vi "Subtask 1.vi"() -> ()   [LabVIEW 2016, in "Test.lvrbt"]
uses:
  Test.lvrbt
  <vilib>/NXT/Block Support/NXT_OutputPort.ctl
  <vilib>/NXT/Block Support/NXT_InputPort.ctl
  <vilib>/NXT/Dual Mode Library/Motors/ResetMotor.vi
  <vilib>/NXT/Dual Mode Library/Waits/Wait_Num(msec).vi
  <vilib>/NXT/Dual Mode Library/Display/drawText.vi
  <vilib>/NXT/Dual Mode Library/Sensors/EV3_Color_Reflect.vi
  <vilib>/NXT/Dual Mode Library/Sensors/Touch_Pressed.vi
  <vilib>/NXT/Dual Mode Library/Sensors/EV3_Ultrasonic_CM.vi
  <vilib>/NXT/Dual Mode Library/Motors/Rotation.vi
  <vilib>/NXT/NXTIO Xnodes/NXTIONodeSubVIs/NXTMoveMotors.vi
  <vilib>/NXT/NXTIO Xnodes/NXTIONodeSubVIs/NXTMotorRunDistance.vi
  <vilib>/NXT/Dual Mode Library/Display/drawNumber.vi
  <vilib>/NXT/NXTIO Xnodes/NXTIONodeSubVIs/NXTMotorSteeringOn.vi
  <vilib>/NXT/NXTIO Xnodes/AddressXNode/NXTIOAddress.xnode
  <vilib>/NXT/Subs/LVHSConnector.ctl
  <vilib>/NXT/NXTIO Xnodes/NXTIOXNode/NXTIO.xnode
  <vilib>/NXT/LegoClasses/BrickReference/BrickReference.lvclass
panel:
  out "kD":dbl(graph)
  out "kI":dbl(graph)
  out "kP":sgl(graph)
  out "Combined":dbl(graph)
  out "Power Sum":dbl
  out "power":dbl
  out "rotation":dbl
  out "button":bool
  out "Distance":dbl
  out "Box Number":dbl
  out "Zone Detector":dbl
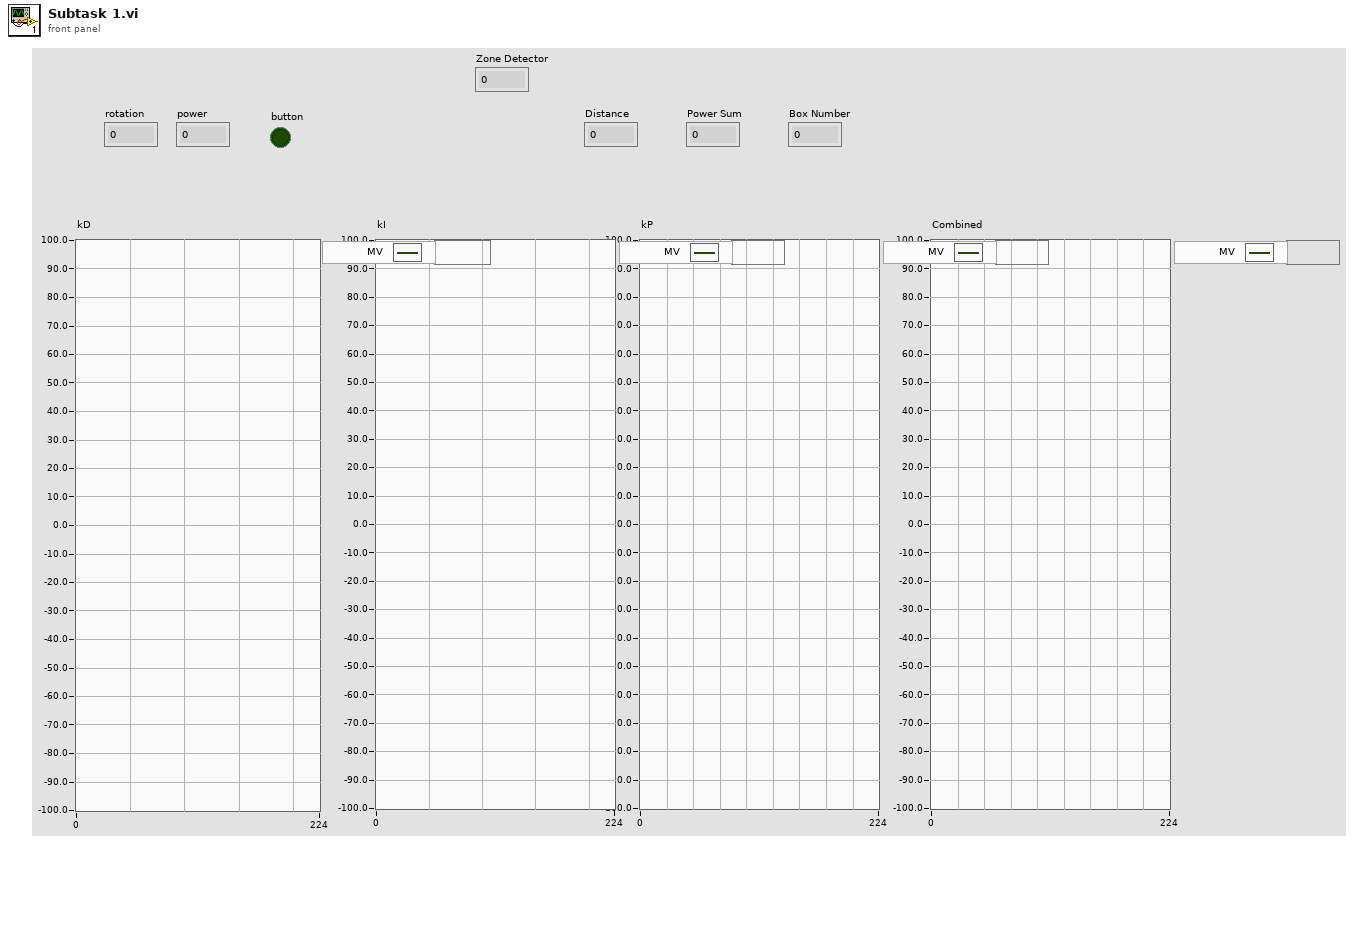
[diagram p1: front panel]
types:
  T1 = typedef "NXT_OutputPort.ctl" = u8
  T2 = typedef "NXT_InputPort.ctl" = u32
  T3 = typedef "LVHSConnector.ctl" = refnum<class "BrickReference.lvclass">
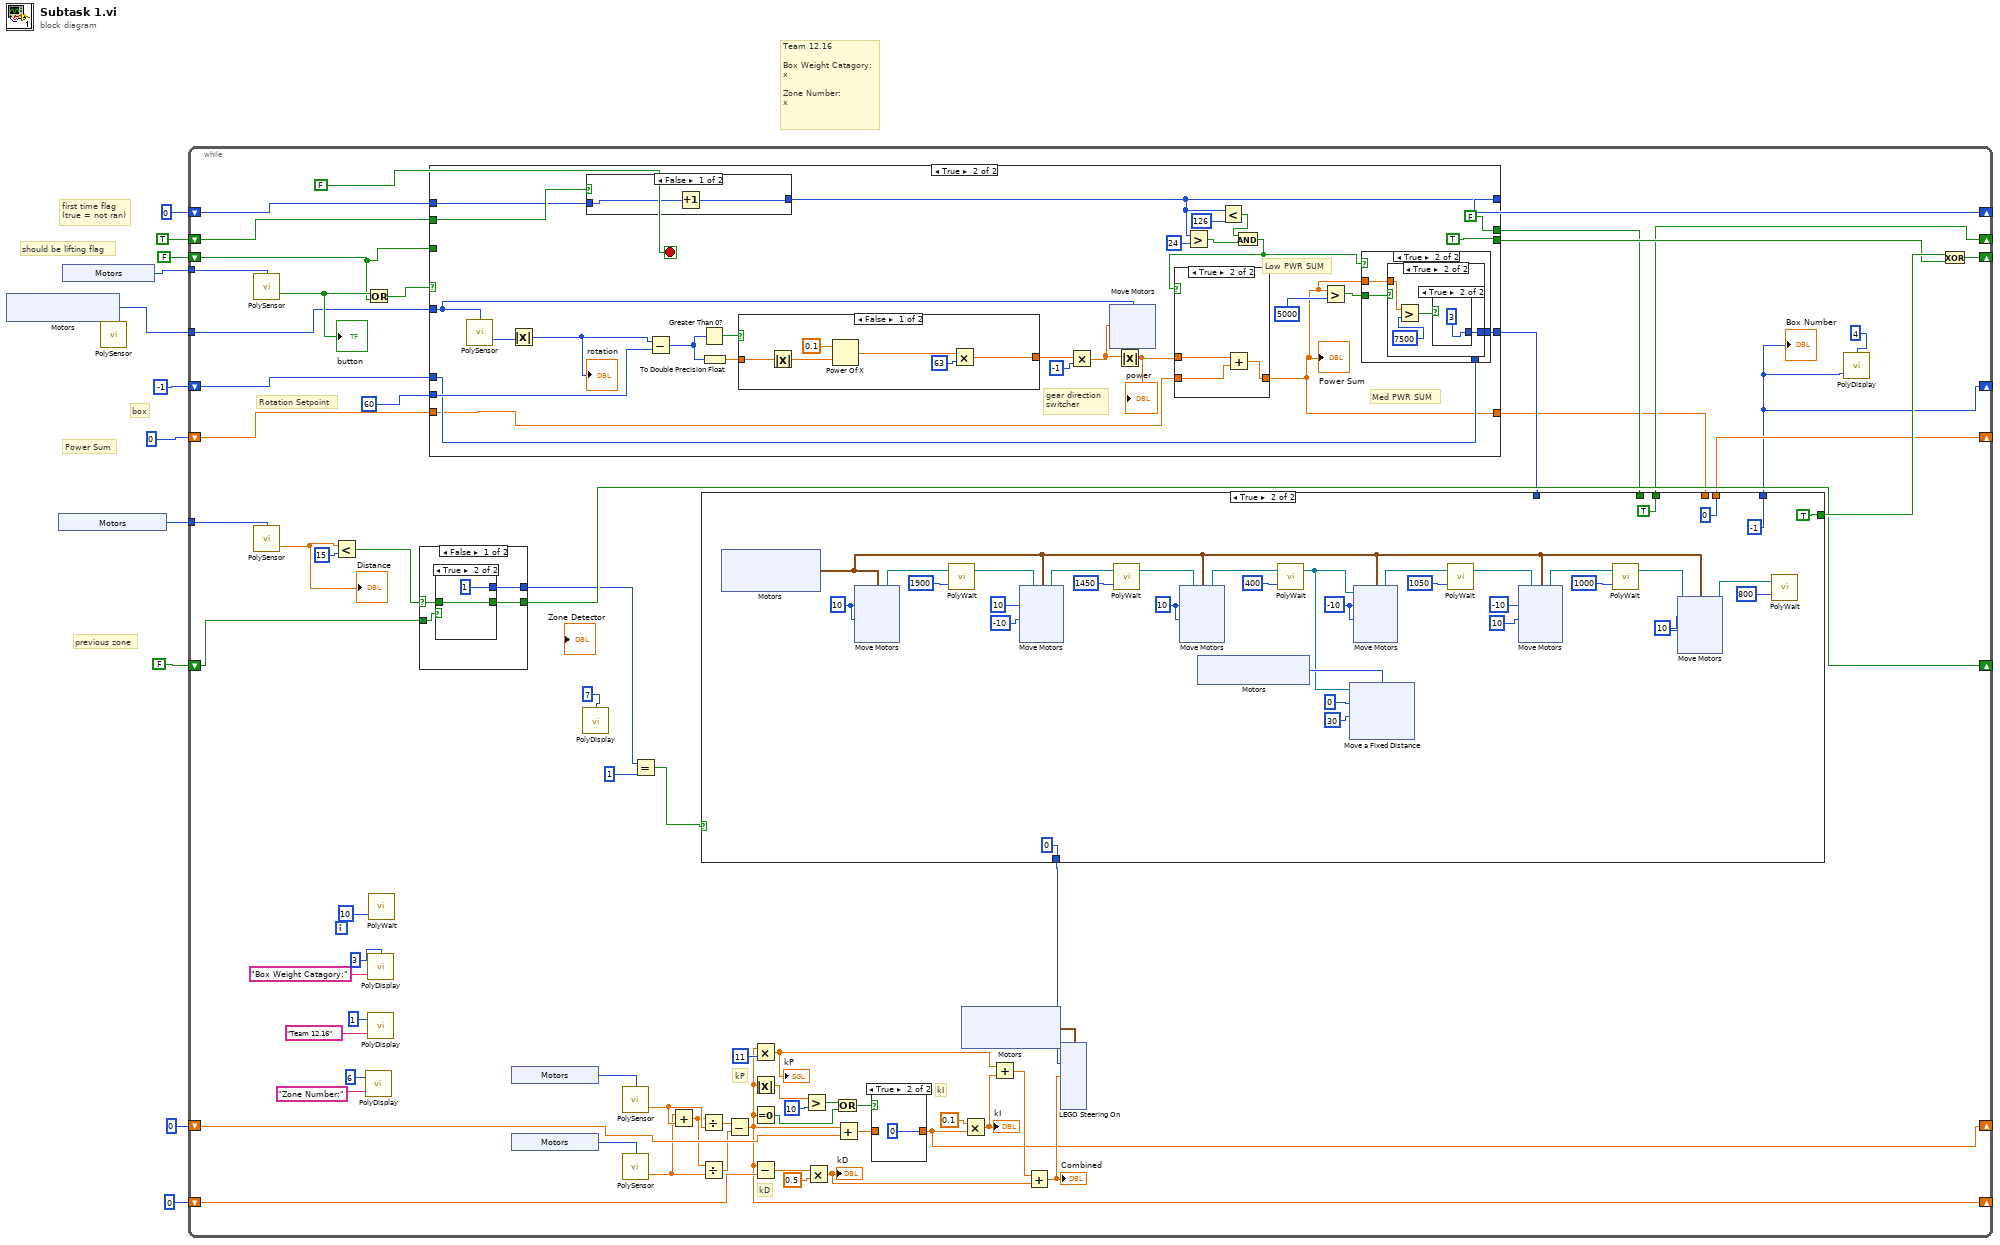
[diagram p0: block diagram]
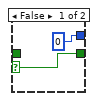
[diagram p2: hidden frame]
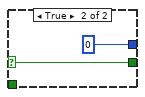
[diagram p3: hidden frame]
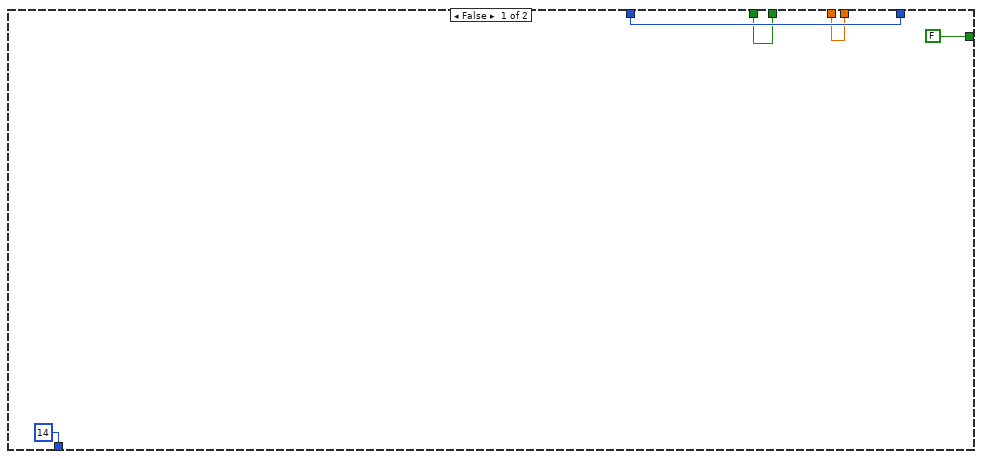
[diagram p4: hidden frame]
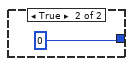
[diagram p6: hidden frame]
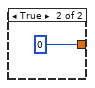
[diagram p8: hidden frame]
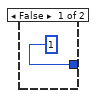
[diagram p10: hidden frame]
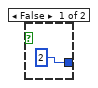
[diagram p11: hidden frame]
diagram:
  # "box"
  # "previous zone"
  # "Team 12.16\n\nBox Weight Catagory:\nx\n\nZone Number:\nx"
  # "should be lifting flag"
  # "first time flag\n(true = not ran)"
  # "Power Sum"
  n1 = xnode "Motors"() -> ("Motor"=w1:T1)
  n2 = xnode "Motors"() -> ("Sensor"=w8:T2)
  n3 = xnode "Motors"() -> ("Sensor"=w7:T2)
  n4 = call-poly <vilib>:"PolySensor.vi"("Port (All Ports)"=w1) -> ()  [unwired: 3 in, 1 out]
  n5 = while {
    shift-right: [w50] -> _
    shift-left: 0 -> [w77]
    shift-right: [w51] -> _
    shift-left: 0 -> [w76]
    tunnel: w1 -> [w32]
    shift-right: [w48] -> _
    shift-left: FALSE -> [w44]
    tunnel: w8 -> [w41]
    tunnel: w7 -> [w42]
    shift-right: [w14] -> _
    shift-left: -1 -> [w40]
    shift-right: [w18] -> _
    shift-left: TRUE -> [w39]
    shift-right: [w16] -> _
    shift-left: 0 -> [w36]
    shift-right: [w34] -> _
    shift-left: u32 0 ("Time (100 msec)") -> [w35]
    shift-right: [w21] -> _
    shift-left: FALSE -> [w22]
    stop <- FALSE stop-if-true
    # "Rotation Setpoint"
    # "kD"
    # "kI"
    # "kP"
    n6 = call-poly <vilib>:"PolySensor.vi"("Port (Port 1)"=w42) -> ("Yes / No"=w53:bool)  [unwired: 2 in, 1 out]
    "button" <- w53
    n7 = call-poly <vilib>:"PolySensor.vi"("Port (Port 1)"=w41) -> ("Centimeters"=w38:sgl)  [unwired: 2 in, 1 out]
    "Distance" <- w38
    n8 = Less?(x=w38, y=15) -> (x < y?=w23:bool)
    n9 = call-poly <vilib>:"PolyDisplay.vi"("Text"="Zone Number:", "Line"=6 ("number")) -> ()  [unwired: 2 in, 1 out]
    n10 = Or(x=w53, y=w44) -> (x .or. y?=w52:bool)
    n11 = call-poly <vilib>:"PolyDisplay.vi"("Text"="Box Weight Catagory:", "Line"=3 ("number")) -> ()  [unwired: 2 in, 1 out]
    n12 = call-poly <vilib>:"PolyDisplay.vi"("Text"="Team 12.16", "Line"=1 ("number")) -> ()  [unwired: 2 in, 1 out]
    n13 = call-poly <vilib>:"PolyWait.vi"("Time (100 msec)"=u32 10) -> ()  [unwired: 3 in, 1 out]
    n14 = case shown="False" w23 {
      selector: w23 -> [w80 w88]
      tunnel: w22 -> [w82 _]
      tunnel: [w81 w88] -> w21
      tunnel: [w79 0] -> w13
      frame False {
        n15 = case shown="True" w82 {
          selector: w82 -> [w84 _]
          tunnel: [w84 w86] -> w81
          tunnel: w80 -> [_ w86]
          tunnel: [0 1] -> w79
          frame False {
          }
          frame True {
          }
        }
      }
      frame True {
      }
    }
    n16 = case shown="True" w52 {
      tunnel: w32 -> [_ w219]
      tunnel: 60 -> [_ w218]
      tunnel: [w192 TRUE] -> w45
      tunnel: w44 -> [w192 _]
      tunnel: [w191 w214] -> w19
      tunnel: w40 -> [w191 w213]
      tunnel: [w190 FALSE] -> w17
      tunnel: w39 -> [w190 w206]
      tunnel: w36 -> [w189 w208]
      tunnel: [w189 w207] -> w15
      tunnel: w35 -> [w188 w205]
      tunnel: [w188 w204] -> w34
      frame False {
      }
      frame True {
        # "gear direction\nswitcher"
        # "Med PWR SUM"
        # "Low PWR SUM"
        n17 = call-poly <vilib>:"PolySensor.vi"("Port (Port A)"=w219) -> ("Angle of Rotation"=w200:i32)  [unwired: 2 in, 1 out]
        n18 = Absolute Value(x=w200) -> (abs(x)=w199:i32)
        "rotation" <- w199
        n19 = case shown="False" w206 {
          tunnel: [w220 u32 0 ("Time (100 msec)")] -> w204
          tunnel: w205 -> [w221 _]
          frame False {
            n20 = Increment(x=w221) -> (x+1=w220:u32)
          }
          frame True {
          }
        }
        n21 = Subtract(x=w199, y=w218) -> (x-y=w212:i32)
        n22 = Greater Than 0?(x=w212) -> (x > 0?=w211:bool)
        n23 = To Double Precision Float(number=w212) -> (double precision float=w210:dbl)
        n24 = case shown="False" w211 {
          tunnel: [w229 0] -> w196
          tunnel: w210 -> [w228 _]
          frame False {
            n25 = Absolute Value(x=w228) -> (abs(x)=w227:dbl)
            n26 = Power Of X(1:w227, 2:0.1) -> (0:w230:dbl)
            n27 = Multiply(x=w230, y=63) -> (x*y=w229:dbl)
          }
          frame True {
          }
        }
        n28 = Multiply(x=w196, y=-1) -> (x*y=w195:dbl)
        n29 = xnode "Move Motors"("Power/Speed 1"=w195, "Motors"=w219) -> ()  [unwired: 1 in, 1 out]
        n30 = Absolute Value(x=w195) -> (abs(x)=w198:dbl)
        "power" <- w198
        n31 = Greater?(x=w204, y=24) -> (0:w201:bool)
        n32 = Less?(x=w204, y=126) -> (x < y?=w202:bool)
        n33 = And(x=w202, y=w201) -> (x .and. y?=w193:bool)
        n34 = case shown="True" w193 {
          tunnel: w198 -> [_ w226]
          tunnel: [w223 w225] -> w207
          tunnel: w208 -> [w223 w224]
          frame False {
          }
          frame True {
            n35 = Add(x=w226, y=w224) -> (x+y=w225:dbl)
          }
        }
        "Power Sum" <- w207
        n36 = Greater?(x=w207, y=5000) -> (0:w216:bool)
        n37 = case shown="True" w193 {
          tunnel: w216 -> [_ w244]
          tunnel: [w241 w243] -> w214
          tunnel: w207 -> [_ w242]
          tunnel: w213 -> [w241 _]
          frame False {
          }
          frame True {
            n38 = case shown="True" w244 {
              tunnel: [1 w246] -> w243
              tunnel: w242 -> [_ w248]
              frame False {
              }
              frame True {
                n39 = Greater?(x=w248, y=7500) -> (0:w249:bool)
                n40 = case shown="True" w249 {
                  tunnel: [2 3] -> w246
                  frame False {
                  }
                  frame True {
                  }
                }
              }
            }
          }
        }
      }
    }
    n41 = xnode "Motors"() -> ("Sensor"=w46:T2)
    n42 = xnode "Motors"() -> ("Sensor"=w75:T2)
    n43 = call-poly <vilib>:"PolyDisplay.vi"("Line"=7 ("number")) -> ()  [unwired: 3 in, 1 out]
    n44 = call-poly <vilib>:"PolySensor.vi"("Port (Port 1)"=w46) -> ("Scaled Value"=w74:sgl)  [unwired: 2 in, 1 out]
    n45 = call-poly <vilib>:"PolySensor.vi"("Port (Port 1)"=w75) -> ("Scaled Value"=w73:sgl)  [unwired: 2 in, 1 out]
    n46 = Equal?(x=w13, y=1) -> (x = y?=w37:bool)
    n47 = Add(x=w73, y=w74) -> (x+y=w72:sgl)
    n48 = Divide(x=w72, y=w74) -> (x/y=w71:sgl)
    n49 = Divide(x=w72, y=w73) -> (x/y=w69:sgl)
    n50 = case shown="True" w37 {
      tunnel: [FALSE TRUE] -> w47
      tunnel: [14 0] -> w31
      tunnel: [w91 -1] -> w14
      tunnel: w19 -> [w91 _]
      tunnel: [w90 TRUE] -> w18
      tunnel: w17 -> [w90 _]
      tunnel: [w89 0] -> w16
      tunnel: w15 -> [w89 _]
      frame False {
      }
      frame True {
        w95 = i8 10 ("Power/Speed 2")
        w109 = i8 -10 ("Power/Speed 2")
        w112 = i8 10 ("Power/Speed 2")
        w111 = i8 10 ("Power/Speed 2")
        n51 = xnode "Motors"() -> ("Motor"=w97:cluster{"Port":T1, "Port":T1})
        n52 = xnode "Move Motors"("Power/Speed 2"=w111, "Power/Speed 1"=w111, "Motors"=w97) -> ("NXT/EV3"=w125:T3)  [unwired: 1 in]
        n53 = call-poly <vilib>:"PolyWait.vi"("Time (100 msec)"=u32 1900, "NXT/EV3"=w125) -> ("NXT/EV3"=w121:T3)  [unwired: 2 in]
        n54 = xnode "Move Motors"("Power/Speed 2"=i8 -10, "Power/Speed 1"=i8 10, "Motors"=w97, "NXT/EV3"=w121) -> ("NXT/EV3"=w120:T3)
        n55 = call-poly <vilib>:"PolyWait.vi"("Time (100 msec)"=u32 1450, "NXT/EV3"=w120) -> ("NXT/EV3"=w116:T3)  [unwired: 2 in]
        n56 = xnode "Move Motors"("Power/Speed 2"=w112, "Power/Speed 1"=w112, "Motors"=w97, "NXT/EV3"=w116) -> ("NXT/EV3"=w118:T3)
        n57 = xnode "Motors"() -> ("Motor"=w115:T1)
        n58 = call-poly <vilib>:"PolyWait.vi"("Time (100 msec)"=u32 400, "NXT/EV3"=w118) -> ("NXT/EV3"=w110:T3)  [unwired: 2 in]
        n59 = xnode "Move a Fixed Distance"("Speed 1"=i8 30 ("Power/Speed 2"), "Distance 1"=i8 0 ("Power/Speed 2"), "Motors"=w115, "NXT/EV3"=w110) -> ()  [unwired: 1 out]
        n60 = xnode "Move Motors"("Power/Speed 2"=w109, "Power/Speed 1"=w109, "Motors"=w97, "NXT/EV3"=w110) -> ("NXT/EV3"=w107:T3)
        n61 = call-poly <vilib>:"PolyWait.vi"("Time (100 msec)"=u32 1050, "NXT/EV3"=w107) -> ("NXT/EV3"=w102:T3)  [unwired: 2 in]
        n62 = xnode "Move Motors"("Power/Speed 2"=i8 10, "Power/Speed 1"=i8 -10, "Motors"=w97, "NXT/EV3"=w102) -> ("NXT/EV3"=w105:T3)
        n63 = call-poly <vilib>:"PolyWait.vi"("Time (100 msec)"=u32 1000, "NXT/EV3"=w105) -> ("NXT/EV3"=w94:T3)  [unwired: 2 in]
        n64 = xnode "Move Motors"("Power/Speed 2"=w95, "Power/Speed 1"=w95, "Motors"=w97, "NXT/EV3"=w94) -> ("NXT/EV3"=w96:T3)
        n65 = call-poly <vilib>:"PolyWait.vi"("Time (100 msec)"=u32 800, "NXT/EV3"=w96) -> ()  [unwired: 2 in, 1 out]
      }
    }
    "Box Number" <- w14
    n66 = Subtract(x=w71, y=w69) -> (x-y=w51:sgl)
    n67 = Multiply(x=w51, y=11) -> (x*y=w56:sgl)
    "kP" <- w56
    n68 = Absolute Value(x=w51) -> (abs(x)=w64:sgl)
    n69 = Equal To 0?(x=w51) -> (x = 0?=w66:bool)
    n70 = Subtract(x=w51, y=w76) -> (x-y=w61:sgl)
    n71 = Greater?(x=w64, y=10) -> (0:w63:bool)
    n72 = Multiply(x=w61, y=0.5) -> (x*y=w58:dbl)
    "kD" <- w58
    n73 = Or(x=w63, y=w66) -> (x .or. y?=w65:bool)
    n74 = Add(x=w51, y=w77) -> (x+y=w68:sgl)
    n75 = case shown="True" w65 {
      tunnel: w68 -> [w252 _]
      tunnel: [w252 0] -> w50
      frame False {
      }
      frame True {
      }
    }
    n76 = xnode "Motors"() -> ("Motor"=w20:cluster{"Port":T1, "Port":T1})
    n77 = Multiply(x=0.1, y=w50) -> (x*y=w57:dbl)
    "kI" <- w57
    n78 = Add(x=w56, y=w57) -> (x+y=w59:dbl)
    n79 = Add(x=w59, y=w58) -> (x+y=w55:dbl)
    "Combined" <- w55
    n80 = xnode "LEGO Steering On"("Steering 1"=w55, "Power 1"=w31, "Motors"=w20) -> ()  [unwired: 1 in, 1 out]
    n81 = call-poly <vilib>:"PolyDisplay.vi"("number"=w14, "Line"=4 ("number")) -> ()  [unwired: 2 in, 1 out]
    n82 = Exclusive Or(1:w45, 2:w47) -> (0:w48:bool)
  }
